vi "dfd_nMAC_circAddNwLoad.vi"(0 "initIdx":fxp<+,16,16>, 1 "len":fxp<+,16,16>, 3 "load":bool, 4 "step":fxp<+,16,16>) -> (7 "idxOut":fxp<+,16,16>)   [LabVIEW 2017]
uses:
  <vilib>/rvi/FXPMathLib/basic elements/FxpAddSub/XNode/nifxpmath_AddSub.xnode
  <vilib>/rvi/FXPMathLib/sim/FxpSim.dll
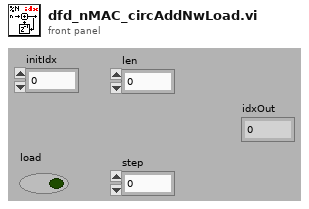
[diagram p1: front panel]
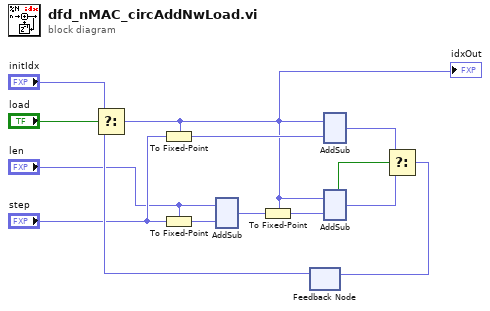
[diagram p0: block diagram]
diagram:
  n1 = To Fixed-Point(fixed-point type="len", number="step") -> (fixed-point=w5:fxp<+,16,16>)
  n2 = xnode "AddSub"("x"="len", "y"=w5) -> ("s"=w6:fxp<+,16,16>)  [unwired: 1 out]
  n3 = feedback #1() -> (w12:fxp<+,16,16>)  [unwired: 1 out]
  n4 = Select(t="initIdx", s="load", f=w12) -> (s? t:f=w1:fxp<+,16,16>)
  "idxOut" <- w1
  n5 = To Fixed-Point(fixed-point type=w1, number="step") -> (fixed-point=w3:fxp<+,16,16>)
  n6 = To Fixed-Point(fixed-point type=w1, number=w6) -> (fixed-point=w2:fxp<+,16,16>)
  n7 = xnode "AddSub"("x"=w1, "y"=w3) -> ("s"=w11:fxp<+,16,16>)  [unwired: 1 out]
  n8 = xnode "AddSub"("x"=w1, "y"=w2) -> ("s"=w10:fxp<+,16,16>, "borrow-out"=w9:bool)
  n9 = Select(t=w11, s=w9, f=w10) -> (s? t:f=w8:fxp<+,16,16>)
  n10 = feedback-in #1(w8) -> ()
